vi "FdxCmdReadEDECounter.vi"(4 "TtLow":u32, 6 "TtHigh":u32, 8 "error in":errorcluster, 9 "EDECounterLow":u32, 10 "EDECounterHigh":u32, 11 "InstrumentHandle":u32) -> (0 "error out":errorcluster, 3 "InstrumentHandle":u32)   [LabVIEW 2020, in "AIM664LV.lvlib"]
doc: "This function is used to read the current value of the EDE reference counter which is used to derive the EDE transmit timestamps. This function is also used to read the IRIG time at which the EDE reference counter was reset to 0."
uses:
  AIM664LV.lvlib
  AFDX_LibraryAdmin/FdxGlobalDllPath.vi
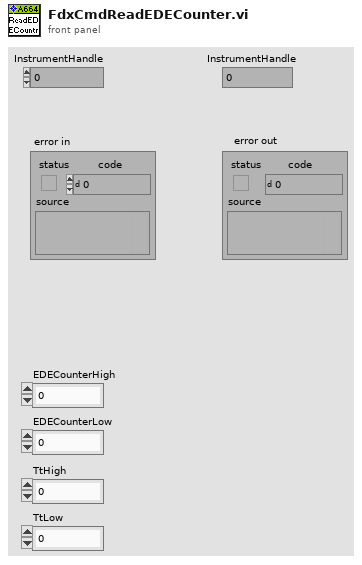
[diagram p1: front panel]
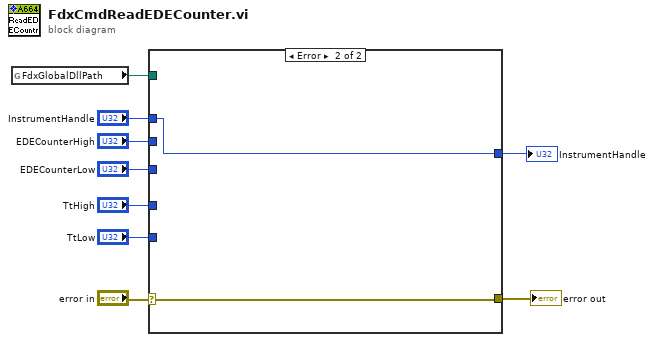
[diagram p0: block diagram]
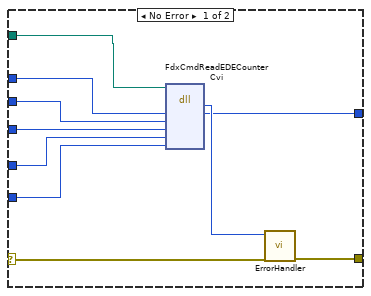
[diagram p2: hidden frame]
diagram:
  n1 = global read "FdxGlobalDllPath.vi" "FdxGlobalDllPath"() -> (w7:path)
  n2 = case shown="Error" "error in" {
    selector: "error in" -> [w18 w21]
    tunnel: [w19 w21] -> w9
    tunnel: w7 -> [w16 _]
    tunnel: [w15 w20] -> w6
    tunnel: "InstrumentHandle" -> [w14 w20]
    tunnel: "EDECounterHigh" -> [w13 _]
    tunnel: "TtLow" -> [w12 _]
    tunnel: "TtHigh" -> [w11 _]
    tunnel: "EDECounterLow" -> [w10 _]
    frame No Error {
      n3 = dll-call lib="aim_fdx.19.dll" fn="FdxCmdReadEDECounterCvi"(path in=w16, "InstrumentHandle"=w14, "EDECounterHigh"=w13, "EDECounterLow"=w10, "TtHigh"=w11, "TtLow"=w12) -> ("status"=w17:i32, "InstrumentHandle"=w15:u32)  [unwired: 2 in, 6 out]
      n4 = call "ErrorHandler.vi"("error in"=w18, "AIM Error"=w17) -> ("error out"=w19:errorcluster)  [unwired: 9 in]
    }
    frame Error {
    }
  }
  "error out" <- w9
  "InstrumentHandle" <- w6
